vi "OR_FreqErrors.vi"(11 "Array":T1[](array[typedef])) -> (3 "ErrorStatus":T1)   [LabVIEW 2018]
uses:
  Controls/Clusts/ErrorStatus.ctl
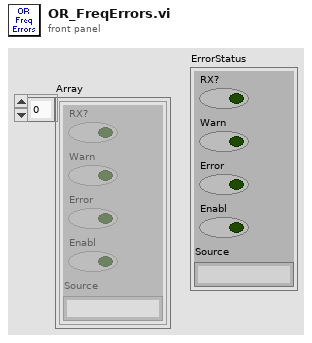
[diagram p1: front panel]
types:
  T1 = typedef "ErrorStatus.ctl" = cluster{"RX?":bool, "Warn":bool, "Error":bool, "Enabl":bool, "Source":string}
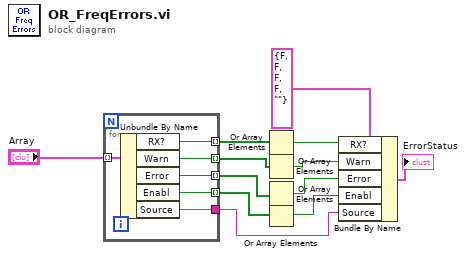
[diagram p0: block diagram]
diagram:
  n1 = for {
    tunnel: "Array" -> [w18] mode=indexing
    tunnel: [w17] -> w10 mode=indexing
    tunnel: [w16] -> w11 mode=indexing
    tunnel: [w15] -> w9 mode=indexing
    tunnel: [w14] -> w3 mode=indexing
    tunnel: [w13] -> w1
    n2 = Unbundle By Name(w18) -> ("RX?"=w16:bool, "Warn"=w17:bool, "Error"=w15:bool, "Enabl"=w14:bool, "Source"=w13:string)
  }
  n3 = Or Array Elements(Boolean array=w11) -> (logical OR=w7:bool)
  n4 = Or Array Elements(Boolean array=w10) -> (logical OR=w6:bool)
  n5 = Or Array Elements(Boolean array=w9) -> (logical OR=w5:bool)
  n6 = Or Array Elements(Boolean array=w3) -> (logical OR=w2:bool)
  n7 = Bundle By Name(cluster=T1 {"RX?"=FALSE, "Warn"=FALSE, "Error"=FALSE, "Enabl"=FALSE, "Source"=""} ("ErrorStatus"), "RX?"=w7, "Warn"=w6, "Error"=w5, "Enabl"=w2, "Source"=w1) -> (→"ErrorStatus":T1)
